vi "FTW-Logger-UpdateFilePath.vi"(0 "FTW Logger":refnum<class "FTW-Logger-Core.lvclass">, 11 "error in":errorcluster) -> (4 "FTW Logger out":refnum<class "FTW-Logger-Core.lvclass">, 15 "error out":errorcluster)   [LabVIEW 2015, in "FTW-Logger-Core.lvclass"]
uses:
  FTW-Logger-Core.lvclass
  FTW-Logger-Core.lvclass/FTW-Logger-Core.ctl
panel:
  # "Inputs"
  # "Outputs"
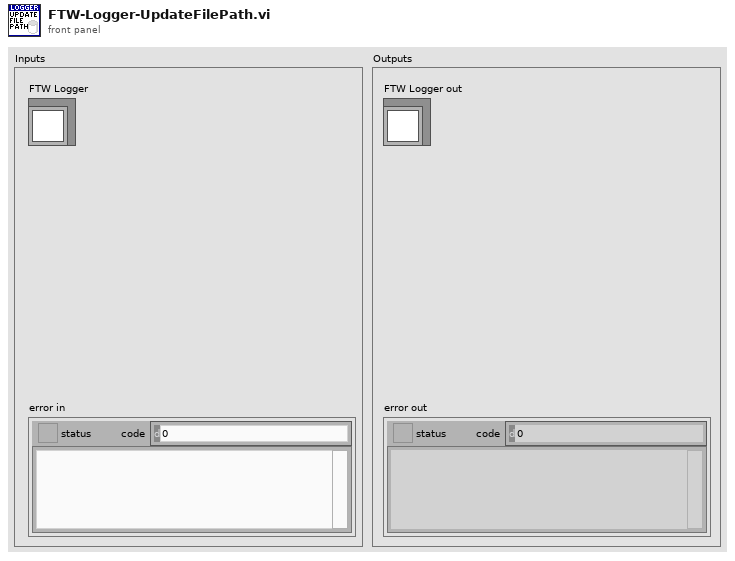
[diagram p1: front panel]
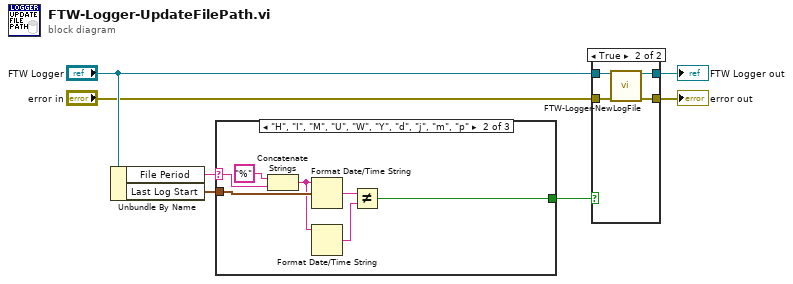
[diagram p0: block diagram]
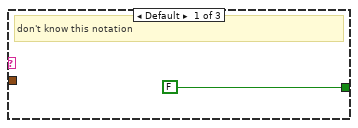
[diagram p3: hidden frame]
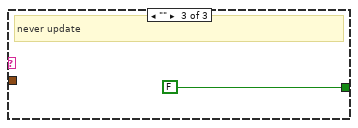
[diagram p4: hidden frame]
diagram:
  n1 = Unbundle By Name("FTW Logger") -> ("File Period"=w6:string, "Last Log Start"=w2:timestamp)
  n2 = case shown="\"H\", \"I\", \"M\", \"U\", \"W\", \"Y\", \"d\", \"j\", \"m\", \"p\"" w6 {
    selector: w6 -> [_ w13 _]
    tunnel: w2 -> [_ w14 _]
    tunnel: [FALSE w15 FALSE] -> w1
    frame Default {
      # "don't know this notation"
    }
    frame "H", "I", "M", "U", "W", "Y", "d", "j", "m", "p" {
      n3 = Concatenate Strings("%" ("string"), w13) -> (w11:string)
      n4 = Format Date/Time String(time format string (%c)=w11, seconds (now)=w14) -> (date/time string=w10:string)  [unwired: 1 in]
      n5 = Format Date/Time String(time format string (%c)=w11) -> (date/time string=w9:string)  [unwired: 2 in]
      n6 = Not Equal?(x=w10, y=w9) -> (x != y?=w15:bool)
    }
    frame "" {
      # "never update"
    }
  }
  n7 = case shown="True" w1 {
    tunnel: "FTW Logger" -> [w17 w22]
    tunnel: [w17 w21] -> w5
    tunnel: "error in" -> [w18 w20]
    tunnel: [w18 w19] -> w3
    frame False {
    }
    frame True {
      n8 = call "FTW-Logger-NewLogFile.vi"("FTW Logger"=w22, "error in"=w20) -> ("FTW Logger out"=w21:refnum<class "FTW-Logger-Core.lvclass">, "error out"=w19:errorcluster)  [unwired: 12 in]
    }
  }
  "error out" <- w3
  "FTW Logger out" <- w5
